vi "Init.vi"(8 "error in (no error)":errorcluster, 11 "FGen PXI Base CFG in":refnum<class "FGen PXI Base CFG.lvclass">) -> (0 "error out":errorcluster, 3 "FGen PXI Base CFG out":refnum<class "FGen PXI Base CFG.lvclass">)   [LabVIEW 2023, in "FGen PXI Base CFG.lvlib" / "FGen PXI Base CFG.lvclass"]
uses:
  FGen PXI Base CFG.lvclass
  FGen PXI Base CFG.lvclass/FGen PXI Base CFG.ctl
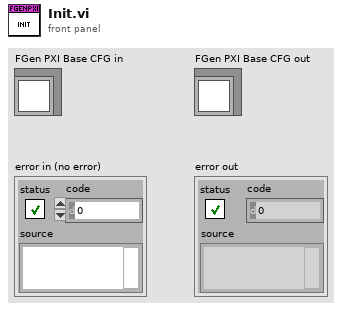
[diagram p1: front panel]
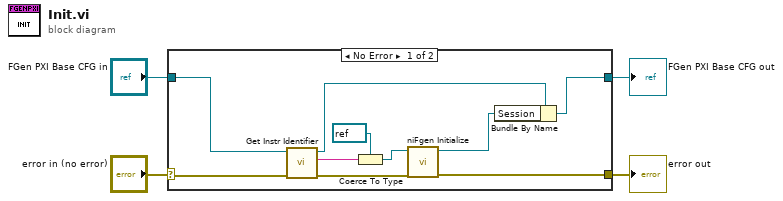
[diagram p0: block diagram]
diagram:
  n1 = case shown="No Error" "error in (no error)" {
    selector: "error in (no error)" -> [w11 w16]
    tunnel: [w13 w16] -> w3
    tunnel: [w12 w15] -> w1
    tunnel: "FGen PXI Base CFG in" -> [w8 w15]
    frame No Error {
      n2 = call-dynamic "Get Instr Identifier.vi"("error in (no error)"=w11, "Configuration Base in"=w8) -> ("error out"=w10:errorcluster, "Instr Identifier"=w9:string, "Configuration Base out"=w7:refnum<class "FGen PXI Base CFG.lvclass">)  [unwired: 7 in]
      n3 = Coerce To Type(0:w9, 1:refnum<k15> refnum ("Resource Name")) -> (2:w5:refnum<k15>)
      n4 = call <instrlib>:"niFgen Initialize.vi"("error in (no error)"=w10, "Resource Name"=w5) -> ("error out"=w13:errorcluster, "Instrument Handle Out"=w14:refnum<k15>)  [unwired: 8 in]
      n5 = Bundle By Name(cluster=w7, "Session"=w14) -> (w12:refnum<class "FGen PXI Base CFG.lvclass">)
    }
    frame Error {
    }
  }
  "error out" <- w3
  "FGen PXI Base CFG out" <- w1
